vi "FromData.vi"(8 "error in (no error)":errorcluster, 10 "Data":string, 11 "Error in":refnum<class "Error.lvclass">) -> (0 "error out":errorcluster, 3 "Error out":refnum<class "Error.lvclass">)   [LabVIEW 2022 SP3, in "Error.lvlib" / "Error.lvclass"]
uses:
  Error.lvclass
  Error.lvclass/Error.ctl
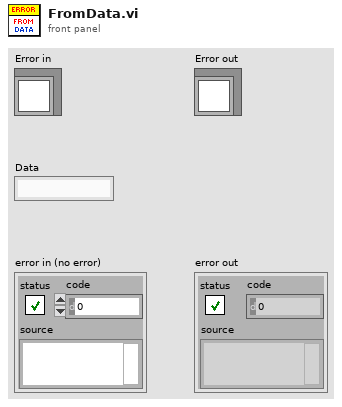
[diagram p1: front panel]
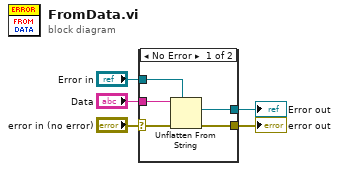
[diagram p0: block diagram]
diagram:
  n1 = case shown="No Error" "error in (no error)" {
    selector: "error in (no error)" -> [w10 w12]
    tunnel: [w9 w12] -> w4
    tunnel: [w6 w11] -> w2
    tunnel: "Error in" -> [w7 w11]
    tunnel: "Data" -> [w8 _]
    frame No Error {
      n2 = Unflatten From String(type=w7, binary string=w8, error in (no error)=w10) -> (value=w6:refnum<class "Error.lvclass">, error out=w9:errorcluster)  [unwired: 2 in, 1 out]
    }
    frame Error {
    }
  }
  "error out" <- w4
  "Error out" <- w2
